vi "CambiarVPC.vi"(1 "Numeric":dbl, 2 "VISA resource name":refnum<visa-resource-name>="COM1") -> (0 "Voltios":string)   [LabVIEW 2011]
doc: "The Advanced Serial Read and Write example performs a Serial Port Read, a Serial Port Write, or a combination of these actions while setting some advanced serial features like buffer size, termination characters, and XON/XOFF flow control. The user selects the actions (read or write) on the front panel. If both are selected, the VI will write the data first, read the data and then close the VISA session that is opened to the port. \n\nThe parameters set for the serial port must match the parameters of the connected instrument or device. In this example, the bytes to read parameter specifies the number of bytes that the serial port reads. If there were more bytes at the port than the number specified in bytes to read, those bytes would not be read. Also, if you specify to read more bytes than the number of bytes actually read, you might receive a timeout error message.\n\nINSTRUCTIONS:\n1) Select the serial resource and configuration parameters (baud rate, data bits, parity, stop bits, flow control).\n2) Termination character can be enabled and set. Also, set the required input buffer size prior to running the example.\n3) Select the operations to be performed. \n4) Connect the serial port to your device. If no device is available, perform a loopback test by doing one of the following. Short pins 2 and 3 on a RS-232 cable or short pin 4 to pin 8 and pin 5 to pin 9 on a RS-485/422 cable. \n5) Run the VI to see the data read. (The \"read string\" will match the \"string to write\" if a loopback test was performed.)\n\nThis example exposes several advanced features that you may need for your application. Not all applications need all the features shown in this example. The input buffer size is likely an important setting that you want to control in your application. This example expands upon the flow control option for XON and XOFF, allowing the user to choose those control characters. The timeout parameter has been brought to the front panel so a user can specify the time period the VISA Read will wait for the number of bytes to read before timing out. Also, the user has several controls for the termination character, which is discussed later.\n\nNote that you can press the write and read buttons and change the bytes to read parameters on the fly, while the example is running. However, you must stop the example to change the other configuration parameters after the example has started running, and then run again.\n\nSet the I/O buffer size slightly higher the amount of data you expect to receive. This is very important for applications that don't use flow control, as you may lose characters if the receive buffer overflows.\n\nSetting the timeout period ensures that the operation returns with a timeout error if the operation cannot be performed in the specified time period. \n\nSome devices require a termination character in order to identify the end of command strings. Some devices send a termination character to signify the end of data to be read. \n\nThis example shows how you can end the Read operation once a termination character is detected in the buffer and/or append a termination character at the end of the Write data. To enable the Read to end on a termination character, use the VISA Configure Serial Port or use the VISA Properties Serial End Mode for Reads, Termination Character Enable, and Termination Character. To end the Write with a termination character, use the VISA Properties Serial End Mode for Writes, the Send End Enable, and Termination Character. In this example, the same termination character is used for both the Read and the Write. You can specify two different characters for your application, if desired.\n\nYour application may require specific characters for the XON/XOFF Flow Control. You can specify these characters with the VISA Properties Flow Control XOFF Character and Flow Control XON Character. Note that if the standard XON and XOFF characters are used, then decimal 17 and 19 are unavailable for data values. Remember that using flow control and setting an adequate buffer size allow you to prevent buffer overflows."
uses:
  Control 1.ctl
  Control 2.ctl
  <vilib>/Instr/_visa.llb/VISA Configure Serial Port (Instr).vi
panel:
  out "Comando Final > 1":string
  out "Sumado <0 2":dbl
  out "Comando Final < 2":string
  in  "PC":dbl
  in  "VMin":dbl
  in  "VMax":dbl
  out "Comando Final < 1":string
  out "Comando Final < 0":string
  out "Comando Final > 0":string
  out "Sumado <0":dbl
  out "Sumado >0":dbl
  out "Numero Leido":string
  in  "flow control":u16(ring) items=["None"=0, "XON/XOFF"=1, "RTS/CTS"=2, "DTR/DSR"=4]
  in  "End write with termination character?":bool=TRUE
  in  "Input\nbuffer size":u32=4096
  in  "termination char\n(0xA = '\\n' = LF)":T1=13 format="%.0x"
  in  "End read on termination character?":bool=TRUE
  in  "timeout (ms)":u32=1000
  in  "parity":u16(ring) items=["None", "Odd", "Even", "Mark", "Space"]
  in  "data bits":u16=8 min=5 max=8 step=1
  in  "stop bits":u16(ring)=10 items=["1.0"=10, "1.5"=15, "2.0"=20]
  in  "baud rate":T2=2400
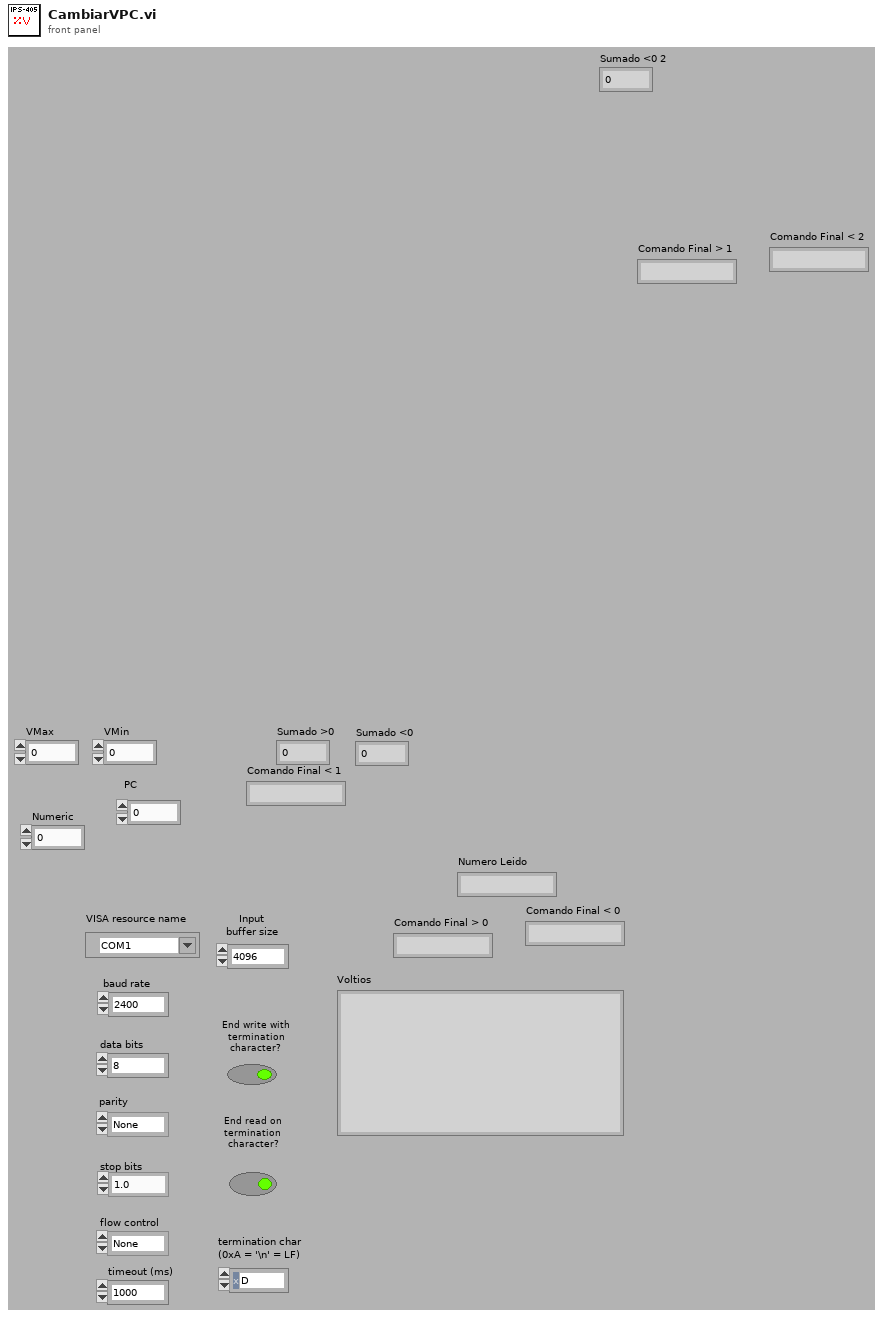
[diagram p1: front panel]
types:
  T1 = typedef "Control 2.ctl" = u8
  T2 = typedef "Control 1.ctl" = u32
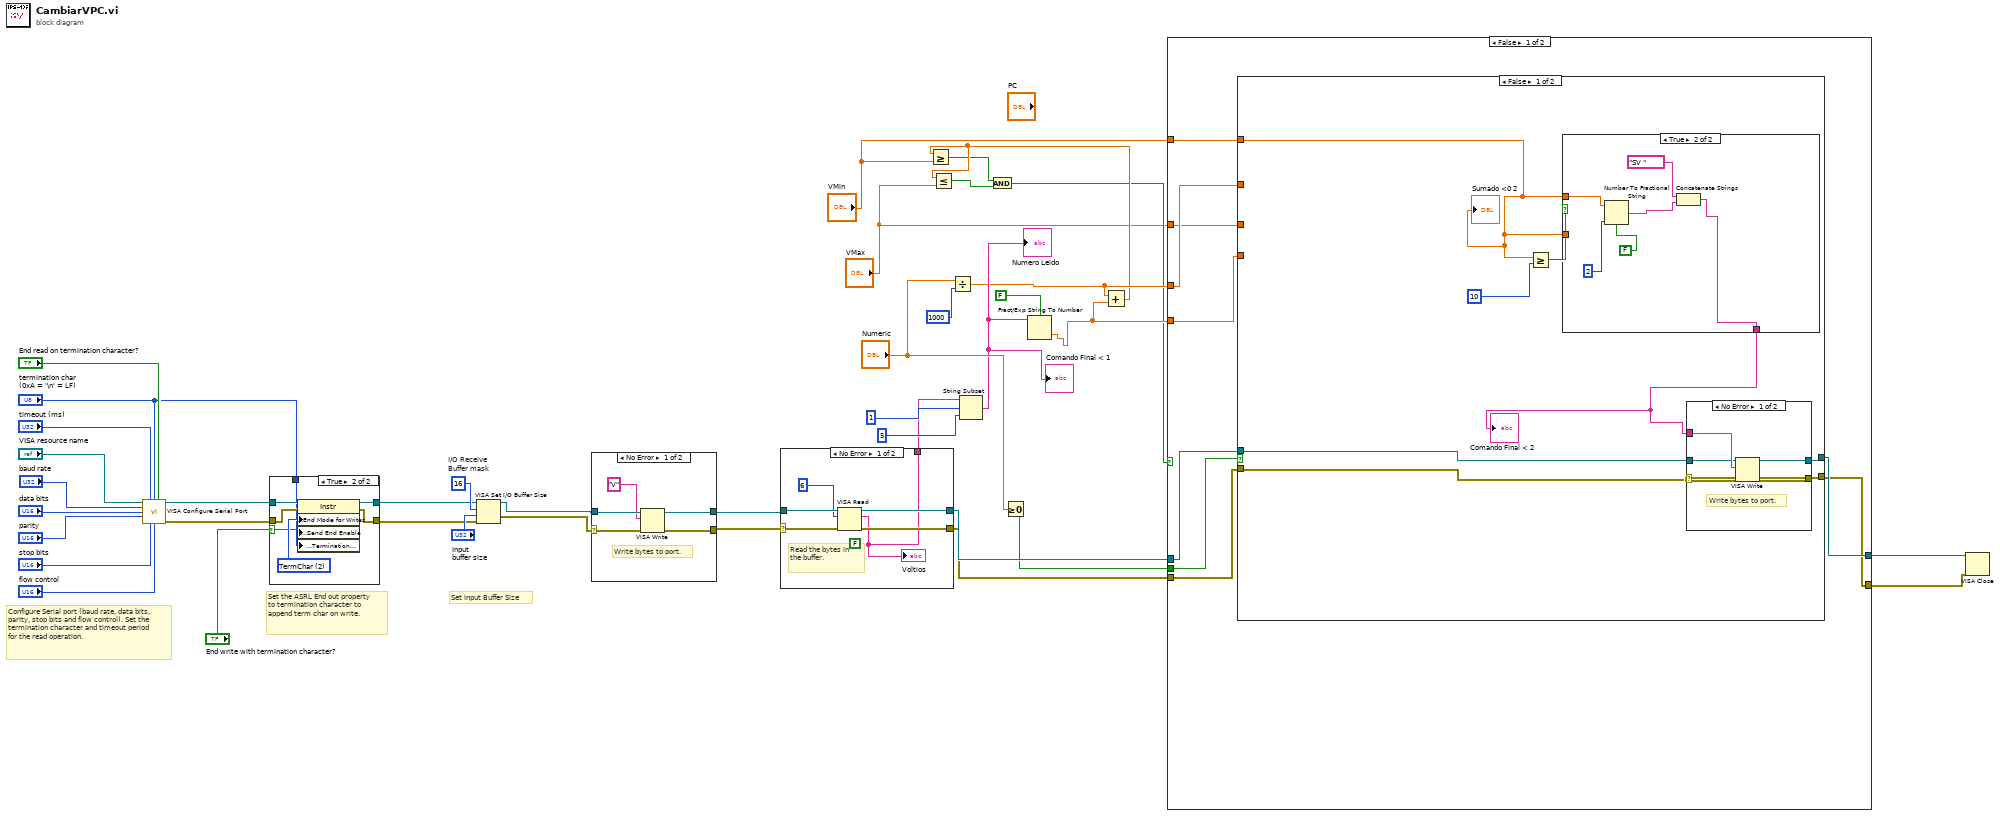
[diagram p0: block diagram]
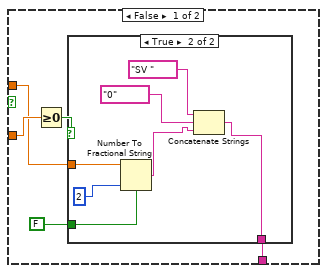
[diagram p2: hidden frame]
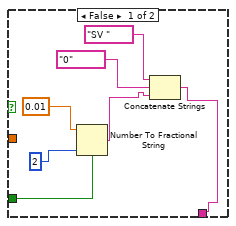
[diagram p3: hidden frame]
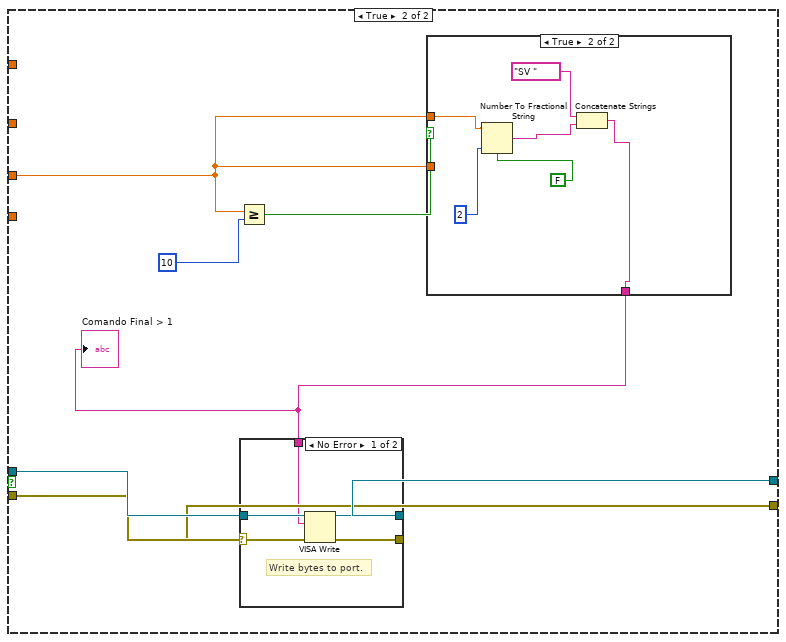
[diagram p5: hidden frame]
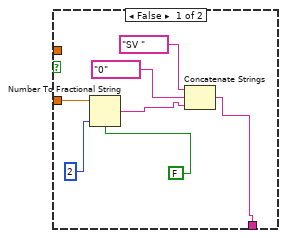
[diagram p6: hidden frame]
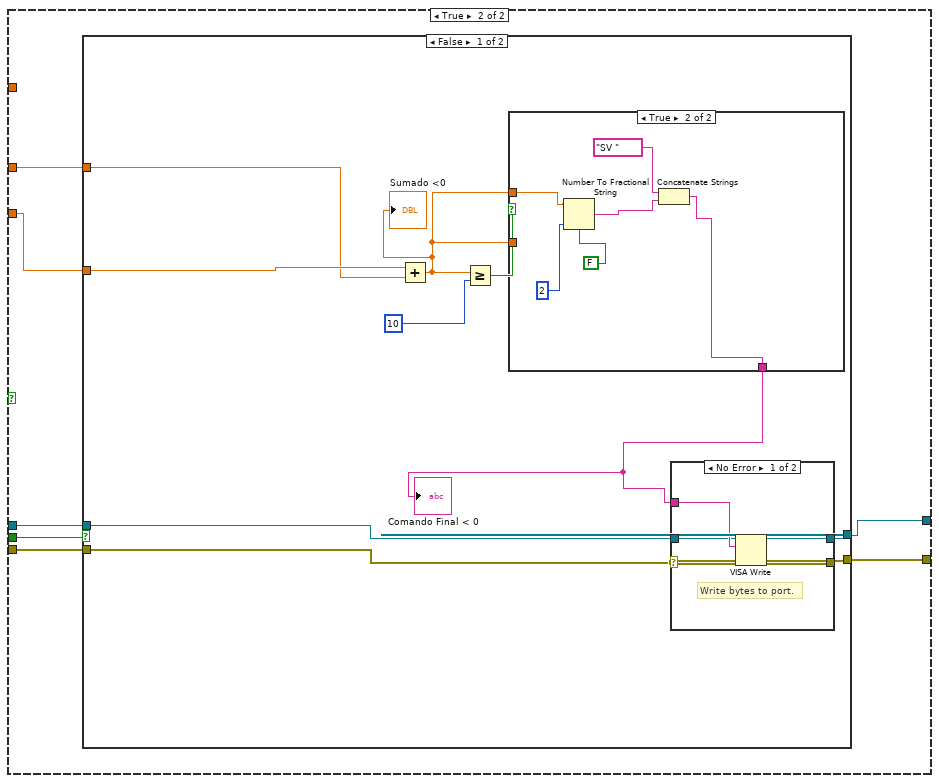
[diagram p8: hidden frame]
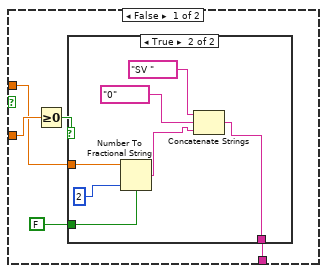
[diagram p9: hidden frame]
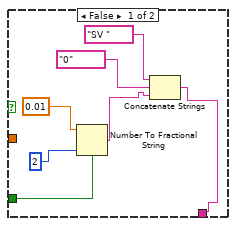
[diagram p10: hidden frame]
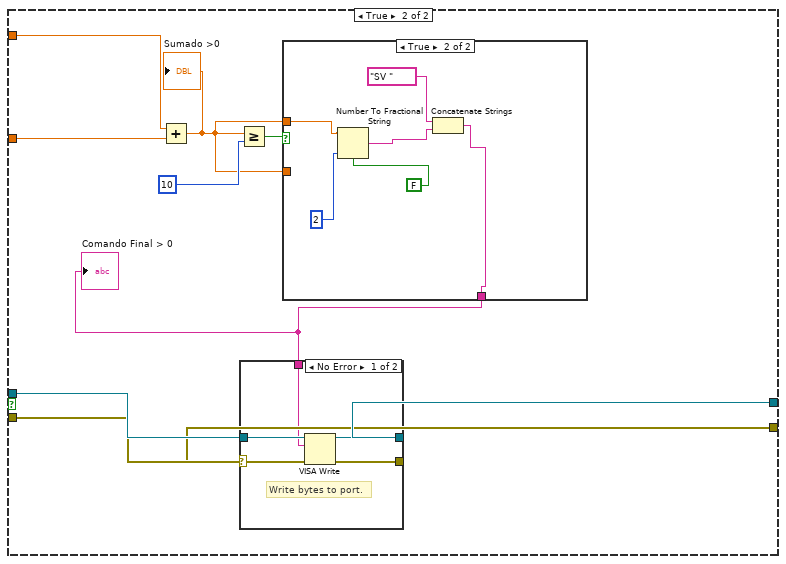
[diagram p12: hidden frame]
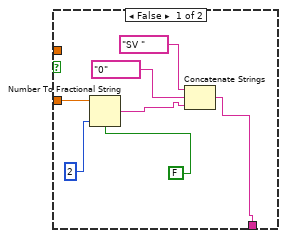
[diagram p13: hidden frame]
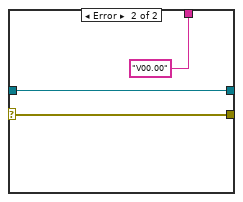
[diagram p15: hidden frame]
diagram:
  w34 = u16 16  # I/O Receive Buffer mask
  # "Configure Serial port (baud rate, data bits, parity, stop bits and flow control). Set the termination character and timeout period for the read operation."
  # "Set Input Buffer Size"
  # "Set the ASRL End out property to termination character to append term char on write."
  n1 = call-poly "VISA Configure Serial Port"("VISA resource name"="VISA resource name", "timeout (10sec)"="timeout (ms)", "termination char\n(0xA = '\\n' = LF)"="termination char\n(0xA = '\\n' = LF)", "Enable Termination\nChar (T)"="End read on termination character?", "baud rate (9600)"="baud rate", "data bits (8)"="data bits", "parity (0:none)"="parity", "stop bits (10: 1 bit)"="stop bits", "flow control (0:none)"="flow control") -> ("VISA resource name out"=w25:refnum<visa-resource-name>, "error out"=w28:errorcluster)  [unwired: 1 in, 4 out]
  n2 = case shown="True" "End write with termination character?" {
    selector: "End write with termination character?" -> [_ w43]
    tunnel: w25 -> [w41 w49]
    tunnel: w28 -> [w42 w48]
    tunnel: [w41 w47] -> w26
    tunnel: [w42 w46] -> w27
    tunnel: "termination char\n(0xA = '\\n' = LF)" -> [_ w44]
    frame False {
    }
    frame True {
      w45 = u16 2 items=["None", "LastBit", "TermChar", "Break"] ("Serial Settings:Serial End Mode for Writes")
      n3 = property class="Instr"(reference=w49, error in=w48, "Serial Settings:End Mode for Writes"=w45, "Message Based Settings:Send End Enable"=w43, "Message Based Settings:Termination Character"=w44) -> (reference out=w47:refnum<visa-resource-name>, error out=w46:errorcluster)
    }
  }
  n4 = VISA Set I/O Buffer Size(VISA resource name=w26, mask (16)=w34, size (4096)="Input\nbuffer size", error in (no error)=w27) -> (VISA resource name out=w24:refnum<visa-resource-name>, error out=w23:errorcluster)
  n5 = case shown="No Error" w23 {
    selector: w23 -> [w52 w56]
    tunnel: [w54 w55] -> w22
    tunnel: [w53 w56] -> w21
    tunnel: w24 -> [w51 w55]
    frame No Error {
      # "Write bytes to port."
      n6 = VISA Write(VISA resource name=w51, write buffer="V", error in (no error)=w52) -> (VISA resource name out=w54:refnum<visa-resource-name>, error out=w53:errorcluster)  [unwired: 1 out]
    }
    frame Error {
    }
  }
  n7 = case "Read bytes from port." shown="No Error" w21 {
    selector: w21 -> [w59 w64]
    tunnel: [w61 w64] -> w19
    tunnel: [w62 w65] -> w20
    tunnel: w22 -> [w60 w65]
    tunnel: [w57 "V00.00"] -> w13
    frame No Error {
      (unwired) FALSE
      # "Read the bytes in the buffer."
      n8 = VISA Read(VISA resource name=w60, byte count=6, error in (no error)=w59) -> (VISA resource name out=w62:refnum<visa-resource-name>, read buffer=w57:string, error out=w61:errorcluster)  [unwired: 1 out]
      "Voltios" <- w57
    }
    frame Error {
      # "Error occurred \nreading Bytes at \nSerial Port"
    }
  }
  n9 = Divide(x="Numeric", y=1000) -> (x/y=w9:dbl)
  n10 = String Subset(string=w13, offset (0)=1, length (rest)=5) -> (substring=w12:string)
  "Numero Leido" <- w12
  "Comando Final < 1" <- w12
  n11 = Greater Or Equal To 0?(x="Numeric") -> (x >= 0?=w18:bool)
  n12 = Fract/Exp String To Number(use system decimal point (T)=FALSE, string=w12) -> (number=w10:dbl)  [unwired: 2 in, 1 out]
  n13 = Add(x=w9, y=w10) -> (x+y=w8:dbl)
  n14 = Greater Or Equal?(x=w8, y="VMin") -> (x >= y?=w7:bool)
  n15 = Less Or Equal?(x=w8, y="VMax") -> (x <= y?=w6:bool)
  n16 = And(x=w7, y=w6) -> (x .and. y?=w5:bool)
  n17 = case shown="False" w5 {
    tunnel: w20 -> [w71 w149]
    tunnel: w19 -> [w72 w148]
    tunnel: w18 -> [w70 w147]
    tunnel: w10 -> [w69 w146]
    tunnel: w9 -> [w68 w145]
    tunnel: [w74 w144] -> w4
    tunnel: [w73 w143] -> w3
    tunnel: "VMax" -> [w67 _]
    tunnel: "VMin" -> [w66 _]
    frame False {
      n18 = case shown="False" w70 {
        tunnel: w71 -> [w81 w122]
        tunnel: w72 -> [w80 w121]
        tunnel: [w79 w120] -> w74
        tunnel: [w82 w119] -> w73
        tunnel: w69 -> [_ _]
        tunnel: w68 -> [_ _]
        tunnel: w67 -> [_ w115]
        tunnel: w66 -> [w75 _]
        frame False {
          n19 = Greater Or Equal?(x=w75, y=10) -> (x >= y?=w78:bool)
          n20 = case shown="True" w78 {
            tunnel: w75 -> [w86 _]
            tunnel: w75 -> [w84 w105]
            tunnel: [w87 w103] -> w76
            frame False {
              n21 = Greater Or Equal To 0?(x=w86) -> (x >= 0?=w85:bool)
              n22 = case shown="True" w85 {
                tunnel: [w90 w97] -> w87
                tunnel: w84 -> [_ w96]
                tunnel: FALSE -> [w88 w95]
                frame False {
                  n23 = Number To Fractional String(use system decimal point (T)=w88, number=0.01, precision (6)=2) -> (F-format string=w93:string)  [unwired: 1 in]
                  n24 = Concatenate Strings("SV ", "0", w93) -> (w90:string)
                }
                frame True {
                  n25 = Number To Fractional String(use system decimal point (T)=w95, number=w96, precision (6)=2) -> (F-format string=w100:string)  [unwired: 1 in]
                  n26 = Concatenate Strings("SV ", "0", w100) -> (w97:string)
                }
              }
            }
            frame True {
              n27 = Number To Fractional String(use system decimal point (T)=FALSE, number=w105, precision (6)=2) -> (F-format string=w106:string)  [unwired: 1 in]
              n28 = Concatenate Strings("SV ", w106) -> (w103:string)
            }
          }
          "Comando Final < 2" <- w76
          n29 = case shown="No Error" w80 {
            selector: w80 -> [w110 w114]
            tunnel: [w112 w113] -> w79
            tunnel: [w111 w114] -> w82
            tunnel: w76 -> [w109 _]
            tunnel: w81 -> [w108 w113]
            frame No Error {
              # "Write bytes to port."
              n30 = VISA Write(VISA resource name=w108, write buffer=w109, error in (no error)=w110) -> (VISA resource name out=w112:refnum<visa-resource-name>, error out=w111:errorcluster)  [unwired: 1 out]
            }
            frame Error {
            }
          }
          "Sumado <0 2" <- w75
        }
        frame True {
          n31 = Greater Or Equal?(x=w115, y=10) -> (x >= y?=w117:bool)
          n32 = case shown="True" w117 {
            tunnel: w115 -> [w126 _]
            tunnel: w115 -> [_ w133]
            tunnel: [w124 w131] -> w116
            frame False {
              n33 = Number To Fractional String(use system decimal point (T)=FALSE, number=w126, precision (6)=2) -> (F-format string=w128:string)  [unwired: 1 in]
              n34 = Concatenate Strings("SV ", "0", w128) -> (w124:string)
            }
            frame True {
              n35 = Number To Fractional String(use system decimal point (T)=FALSE, number=w133, precision (6)=2) -> (F-format string=w134:string)  [unwired: 1 in]
              n36 = Concatenate Strings("SV ", w134) -> (w131:string)
            }
          }
          "Comando Final > 1" <- w116
          n37 = case shown="No Error" w121 {
            selector: w121 -> [w138 w142]
            tunnel: [w140 w141] -> w120
            tunnel: [w139 w142] -> w119
            tunnel: w122 -> [w137 w141]
            tunnel: w116 -> [w136 _]
            frame No Error {
              # "Write bytes to port."
              n38 = VISA Write(VISA resource name=w137, write buffer=w136, error in (no error)=w138) -> (VISA resource name out=w140:refnum<visa-resource-name>, error out=w139:errorcluster)  [unwired: 1 out]
            }
            frame Error {
            }
          }
        }
      }
    }
    frame True {
      n39 = case shown="False" w147 {
        tunnel: w149 -> [w158 w201]
        tunnel: w148 -> [w157 w200]
        tunnel: [w156 w199] -> w144
        tunnel: [w159 w198] -> w143
        tunnel: w145 -> [w151 w196]
        tunnel: w146 -> [w152 w197]
        frame False {
          n40 = Add(x=w152, y=w151) -> (x+y=w153:dbl)
          "Sumado <0" <- w153
          n41 = Greater Or Equal?(x=w153, y=10) -> (x >= y?=w155:bool)
          n42 = case shown="True" w155 {
            tunnel: w153 -> [w163 _]
            tunnel: w153 -> [w161 w182]
            tunnel: [w164 w180] -> w150
            frame False {
              n43 = Greater Or Equal To 0?(x=w163) -> (x >= 0?=w162:bool)
              n44 = case shown="True" w162 {
                tunnel: [w167 w174] -> w164
                tunnel: w161 -> [_ w173]
                tunnel: FALSE -> [w165 w172]
                frame False {
                  n45 = Number To Fractional String(use system decimal point (T)=w165, number=0.01, precision (6)=2) -> (F-format string=w170:string)  [unwired: 1 in]
                  n46 = Concatenate Strings("SV ", "0", w170) -> (w167:string)
                }
                frame True {
                  n47 = Number To Fractional String(use system decimal point (T)=w172, number=w173, precision (6)=2) -> (F-format string=w177:string)  [unwired: 1 in]
                  n48 = Concatenate Strings("SV ", "0", w177) -> (w174:string)
                }
              }
            }
            frame True {
              n49 = Number To Fractional String(use system decimal point (T)=FALSE, number=w182, precision (6)=2) -> (F-format string=w183:string)  [unwired: 1 in]
              n50 = Concatenate Strings("SV ", w183) -> (w180:string)
            }
          }
          "Comando Final < 0" <- w150
          n51 = case shown="No Error" w157 {
            selector: w157 -> [w187 w191]
            tunnel: [w189 w190] -> w156
            tunnel: [w188 w191] -> w159
            tunnel: w150 -> [w186 _]
            tunnel: w158 -> [w185 w190]
            frame No Error {
              # "Write bytes to port."
              n52 = VISA Write(VISA resource name=w185, write buffer=w186, error in (no error)=w187) -> (VISA resource name out=w189:refnum<visa-resource-name>, error out=w188:errorcluster)  [unwired: 1 out]
            }
            frame Error {
            }
          }
        }
        frame True {
          n53 = Add(x=w196, y=w197) -> (x+y=w193:dbl)
          "Sumado >0" <- w193
          n54 = Greater Or Equal?(x=w193, y=10) -> (x >= y?=w194:bool)
          n55 = case shown="True" w194 {
            tunnel: w193 -> [w205 _]
            tunnel: w193 -> [_ w212]
            tunnel: [w203 w210] -> w192
            frame False {
              n56 = Number To Fractional String(use system decimal point (T)=FALSE, number=w205, precision (6)=2) -> (F-format string=w207:string)  [unwired: 1 in]
              n57 = Concatenate Strings("SV ", "0", w207) -> (w203:string)
            }
            frame True {
              n58 = Number To Fractional String(use system decimal point (T)=FALSE, number=w212, precision (6)=2) -> (F-format string=w213:string)  [unwired: 1 in]
              n59 = Concatenate Strings("SV ", w213) -> (w210:string)
            }
          }
          "Comando Final > 0" <- w192
          n60 = case shown="No Error" w200 {
            selector: w200 -> [w217 w221]
            tunnel: [w219 w220] -> w199
            tunnel: [w218 w221] -> w198
            tunnel: w201 -> [w216 w220]
            tunnel: w192 -> [w215 _]
            frame No Error {
              # "Write bytes to port."
              n61 = VISA Write(VISA resource name=w216, write buffer=w215, error in (no error)=w217) -> (VISA resource name out=w219:refnum<visa-resource-name>, error out=w218:errorcluster)  [unwired: 1 out]
            }
            frame Error {
            }
          }
        }
      }
    }
  }
  n62 = VISA Close(VISA resource name=w4, error in (no error)=w3) -> ()  [unwired: 1 out]
